vi "changeState.vi"(6 "interface object in":refnum<k20>, 8 "error in (no error)":errorcluster, 10 "state":u16(ring)=128 items=["start remote node"=1, "stop remote node"=2, "enter pre-operational"=128, "reset node"=129, "reset communication"=130], 11 "MotorController in":refnum<class "MotorController.lvclass">) -> (0 "error out":errorcluster, 1 "interface object out":refnum<k20>, 3 "MotorController out":refnum<class "MotorController.lvclass">)   [LabVIEW 2018, in "MotorController.lvclass"]
uses:
  MotorController.lvclass
  MotorController.lvclass/MotorController.ctl
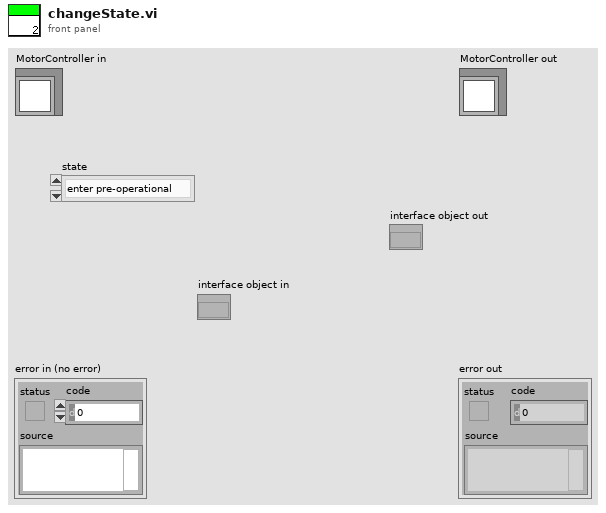
[diagram p1: front panel]
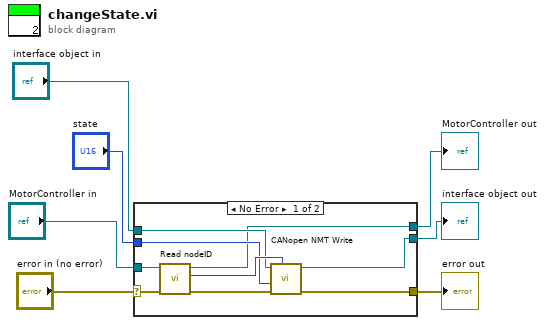
[diagram p0: block diagram]
diagram:
  n1 = case shown="No Error" "error in (no error)" {
    selector: "error in (no error)" -> [w15 w19]
    tunnel: [w9 w19] -> w6
    tunnel: [w8 w18] -> w4
    tunnel: "MotorController in" -> [w16 w18]
    tunnel: "state" -> [w12 _]
    tunnel: "interface object in" -> [w11 w17]
    tunnel: [w10 w17] -> w1
    frame No Error {
      n2 = call "Read nodeID.vi"("error in (no error)"=w15, "MotorController in"=w16) -> ("error out"=w13:errorcluster, "nodeID"=w14:u8, "MotorController out"=w8:refnum<class "MotorController.lvclass">)  [unwired: 7 in]
      n3 = call <vilib>:"CANopen NMT Write.vi"("node-ID (0)"=w14, "error in (no error)"=w13, "command"=w12, "interface object in"=w11) -> ("error out"=w9:errorcluster, "interface object out"=w10:refnum<k20>)  [unwired: 6 in]
    }
    frame Error {
    }
  }
  "error out" <- w6
  "MotorController out" <- w4
  "interface object out" <- w1
